vi "Motor feedback Speed VFD.vi"(8 "error In":errorcluster) -> (0 "error out":errorcluster, 3 "Motor feedback\nspeed":dbl format="%#_13g")   [LabVIEW 2026, in "VFD Library.lvlib"]
uses:
  VFD Library.lvlib
  Private/State Selection FGV.ctl
panel:
  out "Registers":u16[](array[numeric])
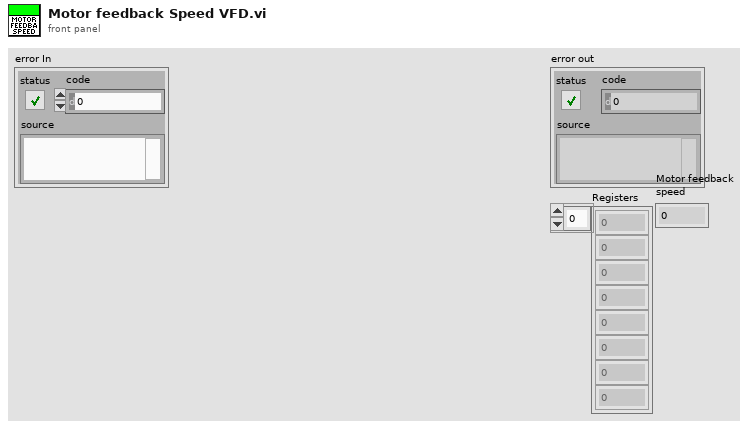
[diagram p1: front panel]
types:
  T1 = typedef "State Selection FGV.ctl" = enum16{"Initilize", "Write Reg", "Write Multiple Reg", "Read Reg", "Write Coil", "Read Coil", "Reset", "Close"}
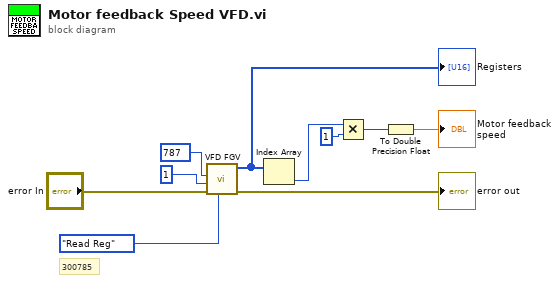
[diagram p0: block diagram]
diagram:
  # "300785"
  n1 = call "VFD FGV.vi"("State"=State_Selection_FGV."Read Reg", "error In"="error In", "value"=u16 1, "address"=u16 787) -> ("error out"=→"error out":errorcluster, "Registers"=w5:u16[])  [unwired: 5 in, 1 out]
  "Registers" <- w5
  n2 = Index Array(array=w5) -> (element=w4:u16)  [unwired: 1 in]
  n3 = Multiply(x=w4, y=u16 1) -> (x*y=w2:u16)
  n4 = To Double Precision Float(number=w2) -> (double precision float=→"Motor feedback\nspeed":dbl)
